vi "Validate Line.vi"(8 "error in (no error)":errorcluster, 10 "Line":T1 {"OPC UA Data Type" items=["Boolean"=1, "SByte"=2, "Byte"=3, "Int16"=4, "UInt16"=5, "Int32"=6, "UInt32"=7, "Int64"=8, "UInt64"=9, "Float"=10, "Double"=11, "String"=12, "DateTime"=13, "ByteString"=15, "Array of Boolean"=101, "Array of SByte"=102, "Array of Byte"=103, "Array of Int16"=104, "Array of UInt16"=105, "Array of Int32"=106, "Array of UInt32"=107, "Array of Int64"=108, "Array of UInt64"=109, "Array of Float"=110, "Array of Double"=111, "Array of String"=112, "Array of DateTime"=113, "Array of ByteString"=115]}, 11 "OPC UA runtime in":refnum<class "OPC UA Client runtime.lvclass">) -> (0 "error out":errorcluster)   [LabVIEW 2014, in "OPC UA Client runtime.lvclass"]
doc: "OPC UA client read/write functions will not return errors or warnings if the access level or data type is incorrect. This VI manually checks this configuration and throws error if configuration is not valid.\n\nWorkaround for CARs 630981 and 631356"
uses:
  OPC UA Client runtime.lvclass
  configuration/Line.ctl
  <vilib>/NI/Tag Bus Module Framework/channel/TBM channel.lvclass
  configuration/OPC UA Data Type.ctl
  OPC UA Client runtime.lvclass/OPC UA Client runtime.ctl
  <vilib>/NI/Tag Bus Module Framework/channel/TBM channel.lvclass/TBM channel.ctl
  <vilib>/NI/Tag Bus Module Framework/channel/channel classification.ctl
  <vilib>/Utility/error.llb/Error Cluster From Error Code.vi
  <vilib>/ErrorRing/Error Ring.xnode
  <vilib>/OPCUA/NI OPC UA Client.lvlib
  configuration/OPC UA Client configuration.lvclass
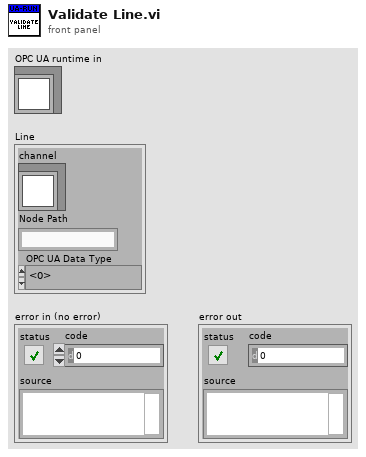
[diagram p1: front panel]
types:
  T1 = typedef "OPC UA Client configuration.lvclass/Line.ctl" = cluster{"channel":refnum<class "TBM channel.lvclass">, "Node Path":string, "OPC UA Data Type":T2}
  T2 = typedef "OPC UA Client configuration.lvclass/OPC UA Data Type.ctl" = u16
  T3 = typedef "TBM channel.lvclass/channel classification.ctl" = enum16{"input data", "output data", "processing parameter", "processing result"}
  T4 = cluster{"name":string, "node type":enum32{"Other", "Folder", "Item/Property"}, "DataType":u32, "access":enum16{"Null", "Read", "Write", "Read&Write"}, "description":string}
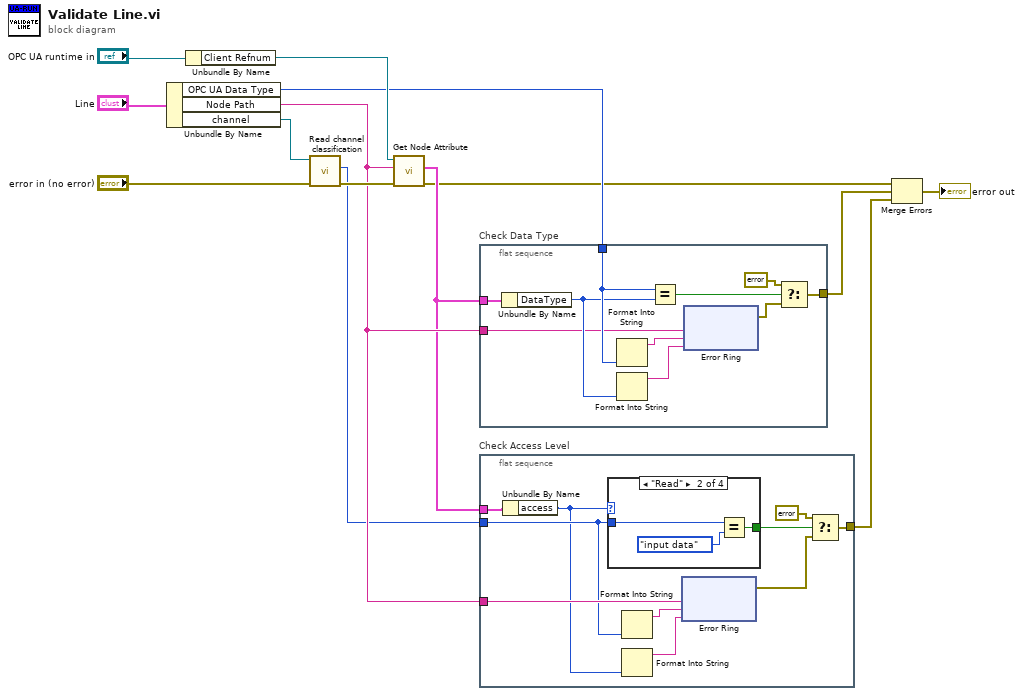
[diagram p0: block diagram]
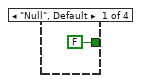
[diagram p2: hidden frame]
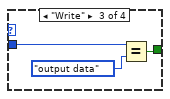
[diagram p3: hidden frame]
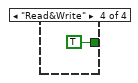
[diagram p4: hidden frame]
diagram:
  n1 = Unbundle By Name("Line") -> ("OPC UA Data Type"=w8:T2, "Node Path"=w7:string, "channel"=w11:refnum<class "TBM channel.lvclass">)
  n2 = Unbundle By Name("OPC UA runtime in") -> ("Client Refnum"=w9:refnum<k21>)
  n3 = call <vilib>:"Read channel classification.vi"("error in"="error in (no error)", "channel in"=w11) -> ("error out"=w10:errorcluster, "channel classification"=w6:T3)  [unwired: 7 in, 1 out]
  n4 = call <vilib>:"Get Node Attribute.vi"("error in (no error)"=w10, "node path"=w7, "OPC UA client refnum in"=w9) -> ("error out"=w4:errorcluster, "node attribute"=w5:T4)  [unwired: 6 in, 1 out]
  n5 = flat-sequence "Check Data Type" {
    tunnel: w8 -> [w22]
    tunnel: w7 -> [w17]
    tunnel: [w16] -> w3
    tunnel: w5 -> [w15]
    frame #0 {
      n6 = Unbundle By Name(w15) -> ("DataType"=w21:u32)
      n7 = Format Into String(w22) -> (resulting string=w20:string)  [unwired: 3 in, 1 out]
      n8 = Format Into String(w21) -> (resulting string=w19:string)  [unwired: 3 in, 1 out]
      n9 = Equal?(x=w22, y=w21) -> (x = y?=w24:bool)
      n10 = xnode "Error Ring"("parameter 0"=w17, "parameter 1"=w20, "parameter 2"=w19) -> ("error out"=w18:errorcluster)
      n11 = Select(t=errorcluster {"status"=FALSE, "code"=0, "source"=""} ("error constant"), s=w24, f=w18) -> (s? t:f=w16:errorcluster)
    }
  }
  n12 = flat-sequence "Check Access Level" {
    tunnel: w7 -> [w41]
    tunnel: w6 -> [w38]
    tunnel: [w36] -> w2
    tunnel: w5 -> [w34]
    frame #0 {
      n13 = Unbundle By Name(w34) -> ("access"=w35:enum16{"Null", "Read", "Write", "Read&Write"})
      n14 = case shown="\"Read\"" w35 {
        tunnel: w38 -> [_ w46 w48 _]
        tunnel: [FALSE w47 w49 TRUE] -> w42
        frame "Null", Default {
        }
        frame "Read" {
          n15 = Equal?(x=w46, y=channel_classification."input data" ("channel classification")) -> (x = y?=w47:bool)
        }
        frame "Write" {
          n16 = Equal?(x=w48, y=channel_classification."output data" ("channel classification")) -> (x = y?=w49:bool)
        }
        frame "Read&Write" {
        }
      }
      n17 = Format Into String(w38) -> (resulting string=w40:string)  [unwired: 3 in, 1 out]
      n18 = Format Into String(w35) -> (resulting string=w39:string)  [unwired: 3 in, 1 out]
      n19 = xnode "Error Ring"("parameter 0"=w41, "parameter 1"=w40, "parameter 2"=w39) -> ("error out"=w37:errorcluster)
      n20 = Select(t=errorcluster {"status"=FALSE, "code"=0, "source"=""} ("error constant"), s=w42, f=w37) -> (s? t:f=w36:errorcluster)
    }
  }
  n21 = Merge Errors(w4, w3, w2) -> (→"error out":errorcluster)
